vi "Encode ABORT Message.vi"(10 "Abort":bool, 11 "Sender ID":string) -> (3 "Abort Message":string[](array[string]))   [LabVIEW 2026, in "TALOS.lvlib" / "Guardian.lvlib" / "Guardian.lvclass"]
uses:
  Guardian.lvclass
  TALOS.lvlib
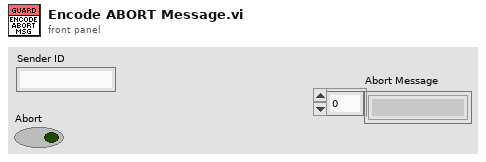
[diagram p1: front panel]
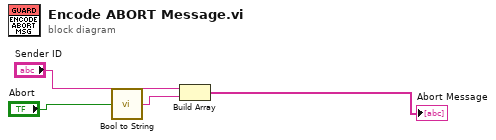
[diagram p0: block diagram]
diagram:
  n1 = call "Bool to String.vi"("Boolean"="Abort") -> ("String"=w2:string)
  n2 = Build Array("Sender ID", w2) -> (→"Abort Message":string[])
